vi "Compute Distance.vi"(6 "Using target width? (t)":bool=TRUE, 8 "Y Image Resolution":i32, 9 "X Image Resolution":i32, 10 "Bounding Box":T1, 11 "Camera Type":enum16{"206", "1011"}(ring)) -> (0 "Angle Offset":dbl(knob) scale=-24.0..24.0, 1 "Target Center (-1 to 1)":cluster{"X":dbl, "Y":dbl}, 2 "Bounding Box (-1 to 1)":T1, 3 "Distance (ft)":dbl)   [LabVIEW 2012]
doc: "Using the camera lens information and the real world width of the target, determine the distance to the target."
panel:
  in  "Camera view angle":dbl[][](array[numeric])=[[36.0, 32.625], [48.0, 43.5]]
  # "Axis 206      Axis M1011"
  # "Vertical"
  # "Horizontal"
  # "Sam's Notes\n\nI added functionality to calculate the angle that \na target is offset horisontally (angle the camera would\nhave to rotate to bring the target to the horizontal center)\n\nI also added the functionality to calculate using the target height instead of width so that if you're camera is at the same height as the target you can calculate distance even from an angle to the side."
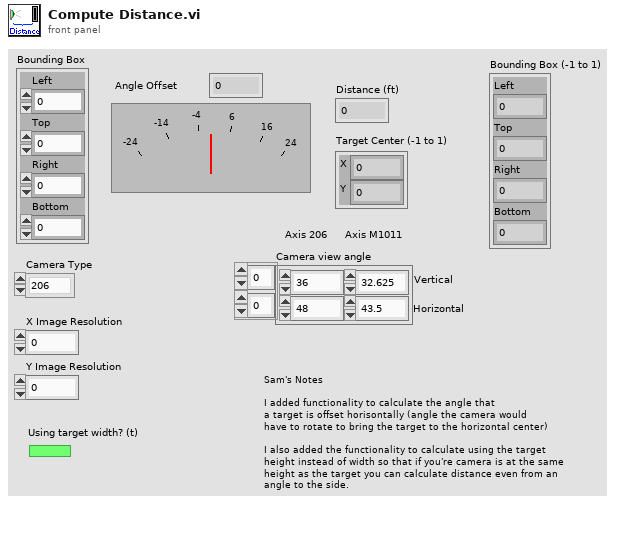
[diagram p1: front panel]
types:
  T1 = cluster{"Left":dbl, "Top":dbl, "Right":dbl, "Bottom":dbl}
  T2 = cluster{"X Image Resolution":i32, "X Image Resolution":i32, "Y Image Resolution":i32, "Y Image Resolution":i32}
  T3 = cluster{"X Image Resolution":i32, "Y Image Resolution":i32}
  T4 = cluster{"X Image Resolution":dbl, "Y Image Resolution":dbl}
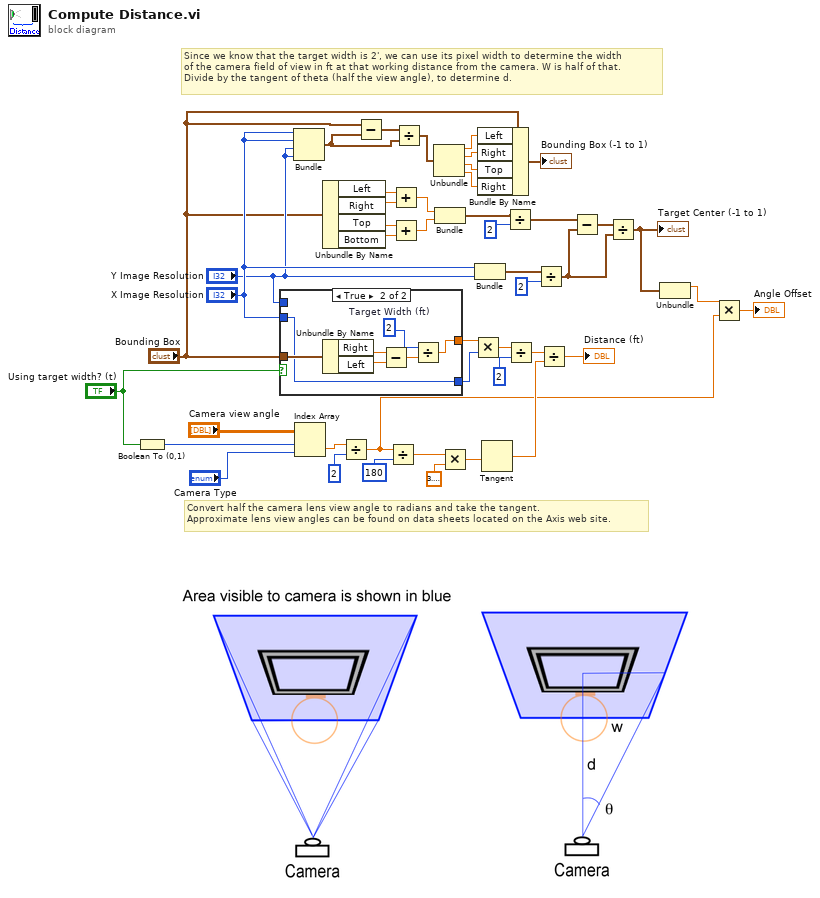
[diagram p0: block diagram]
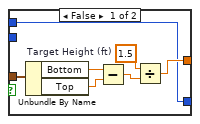
[diagram p2: hidden frame]
diagram:
  # "Convert half the camera lens view angle to radians and take the tangent.\nApproximate lens view angles can be found on data sheets located on the Axis web site."
  # "Since we know that the target width is 2', we can use its pixel width to determine the width\nof the camera field of view in ft at that working distance from the camera. W is half of that.\nDivide by the tangent of theta (half the view angle), to determine d."
  n1 = Boolean To (0,1)(Boolean="Using target width? (t)") -> (0, 1=w12:i16)
  n2 = case shown="True" "Using target width? (t)" {
    tunnel: [w49 w56] -> w15
    tunnel: "Bounding Box" -> [w52 w54]
    tunnel: "X Image Resolution" -> [_ w53]
    tunnel: "Y Image Resolution" -> [w46 _]
    tunnel: [w46 w53] -> w16
    frame False {
      w47 = 1.5  # Target Height (ft)
      n3 = Unbundle By Name(w52) -> ("Bottom"=w50:dbl, "Top"=w51:dbl)
      n4 = Subtract(x=w50, y=w51) -> (x-y=w48:dbl)
      n5 = Divide(x=w47, y=w48) -> (x/y=w49:dbl)
    }
    frame True {
      w55 = 2  # Target Width (ft)
      n6 = Unbundle By Name(w54) -> ("Right"=w59:dbl, "Left"=w58:dbl)
      n7 = Subtract(x=w59, y=w58) -> (x-y=w57:dbl)
      n8 = Divide(x=w55, y=w57) -> (x/y=w56:dbl)
    }
  }
  n9 = Bundle("X Image Resolution"="X Image Resolution", "X Image Resolution"="X Image Resolution", "Y Image Resolution"="Y Image Resolution", "Y Image Resolution"="Y Image Resolution") -> (w8:T2)  [unwired: 1 in]
  n10 = Index Array(array="Camera view angle", index (row)=w12, index (col)="Camera Type") -> (element=w42:dbl)
  n11 = Unbundle By Name("Bounding Box") -> ("Left"=w30:dbl, "Right"=w31:dbl, "Top"=w33:dbl, "Bottom"=w32:dbl)
  n12 = Divide(x=w42, y=2) -> (x/y=w17:dbl)
  n13 = Subtract(x="Bounding Box", y=w8) -> (x-y=w9:cluster{dbl, dbl, dbl, dbl})
  n14 = Divide(x=w17, y=180) -> (x/y=w39:dbl)
  n15 = Add(x=w30, y=w31) -> (x+y=w28:dbl)
  n16 = Add(x=w33, y=w32) -> (x+y=w27:dbl)
  n17 = Divide(x=w9, y=w8) -> (x/y=w6:cluster{dbl, dbl, dbl, dbl})
  n18 = Unbundle(w6) -> (w5:dbl, w4:dbl, w3:dbl, w2:dbl)
  n19 = Bundle(w28, w27) -> (w24:cluster{dbl, dbl})  [unwired: 1 in]
  n20 = Multiply(x=w39, y=3.141592653589793) -> (x*y=w40:dbl)
  n21 = Multiply(x=w15, y=w16) -> (x*y=w34:dbl)
  n22 = Bundle("X Image Resolution"="X Image Resolution", "Y Image Resolution"="Y Image Resolution") -> (w26:T3)  [unwired: 1 in]
  n23 = Bundle By Name(cluster="Bounding Box", "Left"=w5, "Right"=w4, "Top"=w3, "Right"=w2) -> (→"Bounding Box (-1 to 1)":T1)
  n24 = Tangent(1:w40) -> (0:w45:dbl)
  n25 = Divide(x=w24, y=2) -> (x/y=w23:cluster{dbl, dbl})
  n26 = Divide(x=w34, y=2) -> (x/y=w36:dbl)
  n27 = Divide(x=w26, y=2) -> (x/y=w21:T4)
  n28 = Divide(x=w36, y=w45) -> (x/y=→"Distance (ft)":dbl)
  n29 = Subtract(x=w23, y=w21) -> (x-y=w22:cluster{dbl, dbl})
  n30 = Divide(x=w22, y=w21) -> (x/y=w20:cluster{dbl, dbl})
  "Target Center (-1 to 1)" <- w20
  n31 = Unbundle(w20) -> (w18:dbl)  [unwired: 1 out]
  n32 = Multiply(x=w18, y=w17) -> (x*y=→"Angle Offset":dbl)
